vi "Start TCP Comms.vi"(8 "error in (no error)":errorcluster, 11 "Guardian in":refnum<class "Guardian.lvclass">) -> (0 "error out":errorcluster, 3 "Guardian out":refnum<class "Guardian.lvclass">)   [LabVIEW 2026, in "TALOS.lvlib" / "Guardian.lvlib" / "Guardian.lvclass"]
uses:
  Guardian.lvclass
  Ancestor/Ancestor/Ancestor.lvclass/Ancestor.ctl
  Support VIs/Generate Error.vi
  FGV/Error Memory/Get Error Description.vi
  Support VIs/Get PC name.vi
  Ancestor/Ancestor/Read ID.vi
  Support VIs/Get Class Name.vi
  <vilib>/Utility/error.llb/Clear Errors.vi
  FGV/Error Memory/Error Memory Core.vi
  <vilib>/AdvancedString/Delimited String to 1D String Array.vi
  <vilib>/AdvancedString/Delimited String to 1D String Array (string).vi
  Support VIs/Circus Root Path.vi
  FGV/Error Memory/Error Crt Lvl checker.vi
  FGV/Error Memory/Error Memory Core.vi/40c8088d-b597-4017-91af-faa98e00292e.vi
  FGV/Error Memory/Error Memory Core.vi/d4a3ab98-063c-4e44-b43d-fbdcfe6c2be2.vi
  Support VIs/Global Constants.vi
  Support VIs/Global Memory.vi
  <vilib>/Utility/LVClass/Get LV Class Name.vi
  Support VIs/Is in Packed Library.vi
  Support VIs/TALOS Root path.vi
  Support VIs/Read CSV worksheet.vi
  <vilib>/Utility/error.llb/General Error Handler.vi
  Support VIs/Error Log.vi
  Ancestor/Ancestor/Ancestor.lvclass
  <vilib>/Comparison/Equal/Equal Functor/Equal Functor.lvclass
  TALOS.lvlib
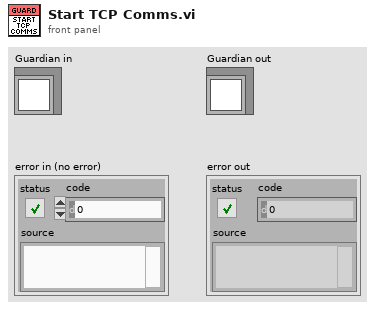
[diagram p1: front panel]
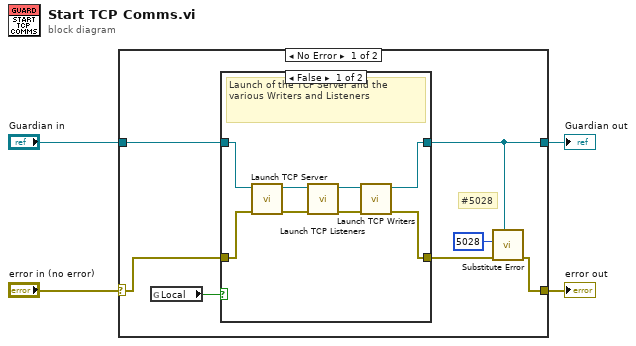
[diagram p0: block diagram]
diagram:
  n1 = case shown="No Error" "error in (no error)" {
    selector: "error in (no error)" -> [w9 w22]
    tunnel: [w7 w22] -> w4
    tunnel: "Guardian in" -> [w10 w23]
    tunnel: [w5 w23] -> w1
    frame No Error {
      # "#5028"
      n2 = global read "Global Constants.vi" "Local"() -> (w11:bool)
      n3 = case shown="False" w11 {
        tunnel: [w12 w20] -> w8
        tunnel: [w14 w21] -> w5
        tunnel: w10 -> [w18 w21]
        tunnel: w9 -> [w19 w20]
        frame False {
          # "Launch of the TCP Server and the various Writers and Listeners"
          n4 = call "Launch TCP Server.vi"("error in (no error)"=w19, "Guardian in"=w18) -> ("error out"=w16:errorcluster, "Guardian out"=w17:refnum<class "Guardian.lvclass">)  [unwired: 8 in]
          n5 = call "Launch TCP Listeners.vi"("error in (no error)"=w16, "Guardian in"=w17) -> ("error out"=w13:errorcluster, "Guardian out"=w15:refnum<class "Guardian.lvclass">)  [unwired: 8 in]
          n6 = call "Launch TCP Writers.vi"("error in (no error)"=w13, "Guardian in"=w15) -> ("error out"=w12:errorcluster, "Guardian out"=w14:refnum<class "Guardian.lvclass">)  [unwired: 8 in]
        }
        frame True {
          # "We are running in locale, no comm.s with the other computers (Kasli included)."
        }
      }
      n7 = call "Substitute Error.vi"("LabVIEW Object"=w5, "error in (no error)"=w8, "Error Code"=5028) -> ("error out"=w7:errorcluster)  [unwired: 8 in]
    }
    frame Error {
    }
  }
  "error out" <- w4
  "Guardian out" <- w1
